vi "TVC_calibration.vi"() -> ()   [LabVIEW 2019]
uses:
  <vilib>/Utility/error.llb/DialogType.ctl
  <vilib>/DAQmx/read.llb/DAQmx Read (Analog 1D DBL NChan 1Samp).vi
  <vilib>/DAQmx/create/channels.llb/DAQmx Create Channel (AI-Voltage-Basic).vi
  <vilib>/DAQmx/configure/timing.llb/DAQmx Timing (Sample Clock).vi
  <vilib>/DAQmx/miscellaneous.llb/DAQmx Fill In Error Info.vi
panel:
  out "data":dbl[](array[numeric]) format="%0.2f"
  out "output variable":sgl
  out "X - Axis":bool
  in  "Y - Axis":tag
  in  "X-Axis":tag
  in  "?":bool
  out "output variable 2":sgl
  out "Y - Axis":bool
  # "Channels"
  # "X- Axis"
  # "Autour: Kaylin Gopal\nTeam: HALE - TVC \n\nCalibration of TVC test Stand"
  # "How To Use:\n\n1. Stuff\n2. More Stuff\n3. Press Start\n4. Calibrate the system"
  # "Y- Axis"
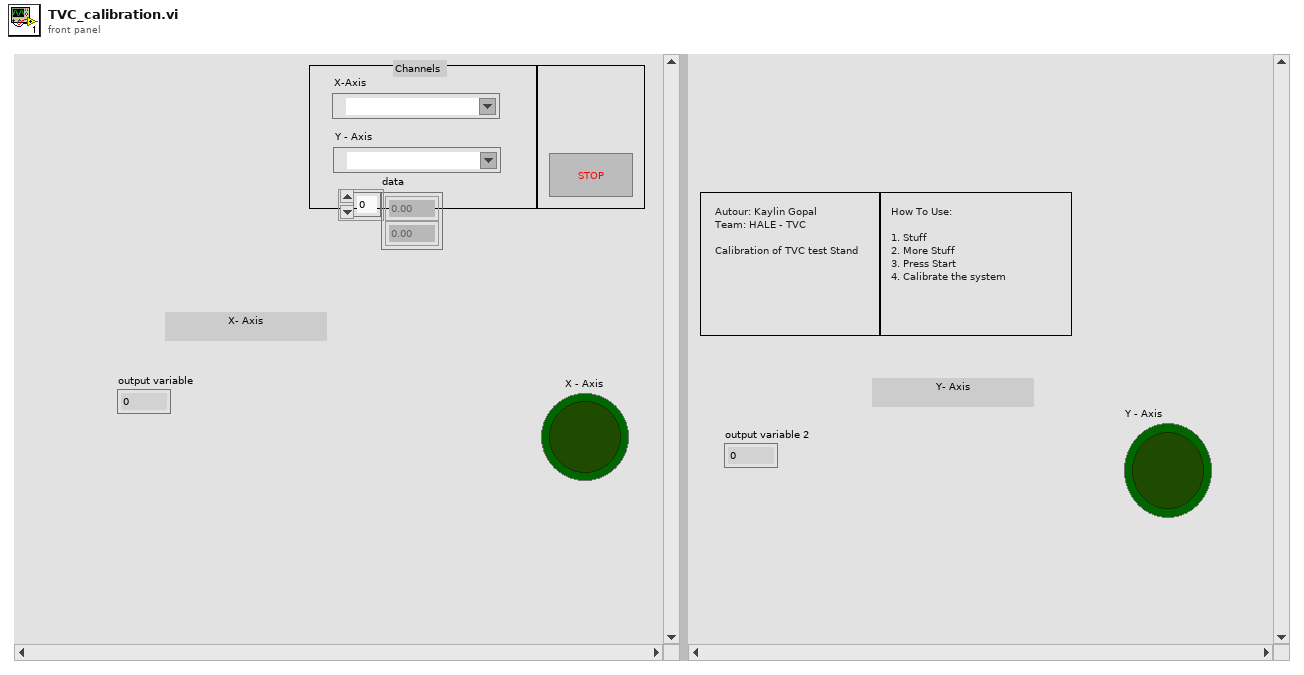
[diagram p1: front panel]
types:
  T1 = typedef "DialogType.ctl" = u16
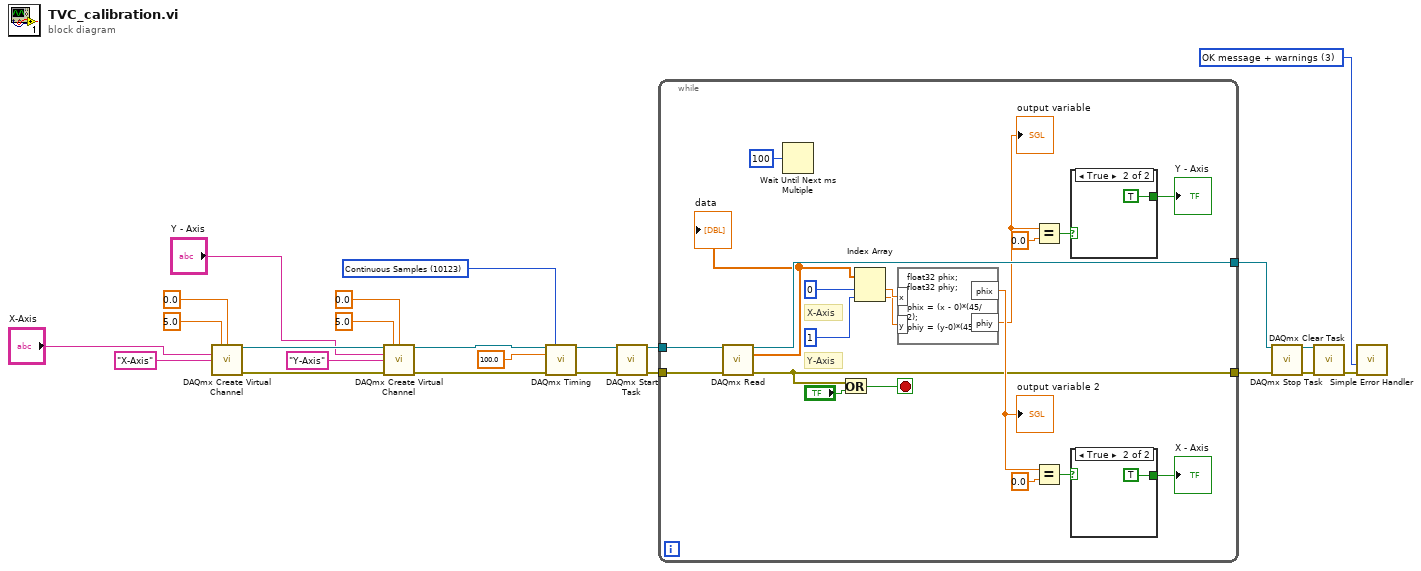
[diagram p0: block diagram]
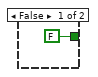
[diagram p2: hidden frame]
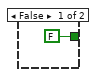
[diagram p3: hidden frame]
diagram:
  w1 = 10123 items=["Finite Samples"=10178, "Continuous Samples"=10123, "Hardware Timed Single Point"=12522] ("sample mode")
  w2 = T1 3 items=["no dialog", "OK message", "continue or stop message", "OK message + warnings", "continue/stop + warnings"] ("type of dialog (OK msg:1)")
  n1 = call-poly <vilib>:"DAQmx Create Virtual Channel.vi"("maximum value"=5.0, "minimum value"=0.0, "physical channels"="X-Axis", "name to assign"="X-Axis") -> ("task out"=w22:refnum<k21>, "error out"=w21:errorcluster)  [unwired: 10 in]
  n2 = call-poly <vilib>:"DAQmx Create Virtual Channel.vi"("task in"=w22, "maximum value"=5.0, "minimum value"=0.0, "physical channels"="Y - Axis", "name to assign"="Y-Axis", "error in"=w21) -> ("task out"=w13:refnum<k21>, "error out"=w14:errorcluster)  [unwired: 8 in]
  n3 = call-poly <vilib>:"DAQmx Timing.vi"("task/channels in"=w13, "sample mode"=w1, "rate"=100.0, "error in"=w14) -> ("task out"=w10:refnum<k21>, "error out"=w11:errorcluster)  [unwired: 10 in]
  n4 = call <vilib>:"DAQmx Start Task.vi"("task/channels in"=w10, "error in"=w11) -> ("task out"=w9:refnum<k21>, "error out"=w8:errorcluster)  [unwired: 12 in]
  n5 = while {
    tunnel: w9 -> [w44]
    tunnel: w8 -> [w43]
    tunnel: [w42] -> w7
    tunnel: [w26] -> w6
    stop <- w28 stop-if-true
    # "Y-Axis"
    # "X-Axis"
    n6 = call-poly <vilib>:"DAQmx Read.vi"("task/channels in"=w44, "error in"=w43) -> ("task out"=w42:refnum<k21>, "data"=w41:dbl[], "error out"=w26:errorcluster)  [unwired: 11 in]
    "data" <- w41
    n7 = Wait Until Next ms Multiple(millisecond multiple=u32 100) -> ()  [unwired: 1 out]
    n8 = Or(x=w26, y="?") -> (x .or. y?=w28:bool)
    n9 = Index Array(array=w41, index #1=0 ("index"), index #2=1 ("index")) -> (element #1=w38:dbl, element #2=w37:dbl)
    n10 = formula code="float32 phix;\nfloat32 phiy;\n\nphix = (x - 0)*(45/2);\nphiy = (y-0)*(45/2);"("x"=w38, "y"=w37) -> ("phix"=w36:sgl, "phiy"=w34:sgl)
    "output variable" <- w34
    "output variable 2" <- w36
    n11 = Equal?(x=w34, y=0.0) -> (x = y?=w29:bool)
    n12 = Equal?(x=w36, y=0.0) -> (x = y?=w32:bool)
    n13 = case shown="True" w29 {
      tunnel: [FALSE TRUE] -> w30
      frame False {
      }
      frame True {
      }
    }
    "Y - Axis" <- w30
    n14 = case shown="True" w32 {
      tunnel: [FALSE TRUE] -> w31
      frame False {
      }
      frame True {
      }
    }
    "X - Axis" <- w31
  }
  n15 = call <vilib>:"DAQmx Stop Task.vi"("task/channels in"=w7, "error in"=w6) -> ("task out"=w5:refnum<k21>, "error out"=w4:errorcluster)  [unwired: 12 in]
  n16 = call <vilib>:"DAQmx Clear Task.vi"("task in"=w5, "error in"=w4) -> ("error out"=w3:errorcluster)  [unwired: 13 in]
  n17 = call <vilib>:"Simple Error Handler.vi"("type of dialog (OK msg:1)"=w2, "error in (no error)"=w3) -> ()  [unwired: 3 in, 5 out]
